vi "ch0 power normalization.vi"(1 "% of max":dbl=0.63, 2 "Gain":fxp<+,32,4>[](array[numeric]), 3 "Wave freq":fxp<+/-,64,32>[](array[numeric])) -> (0 "Array":fxp<+,32,2>[](array[numeric]))   [LabVIEW 2020]
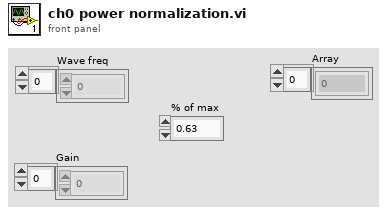
[diagram p1: front panel]
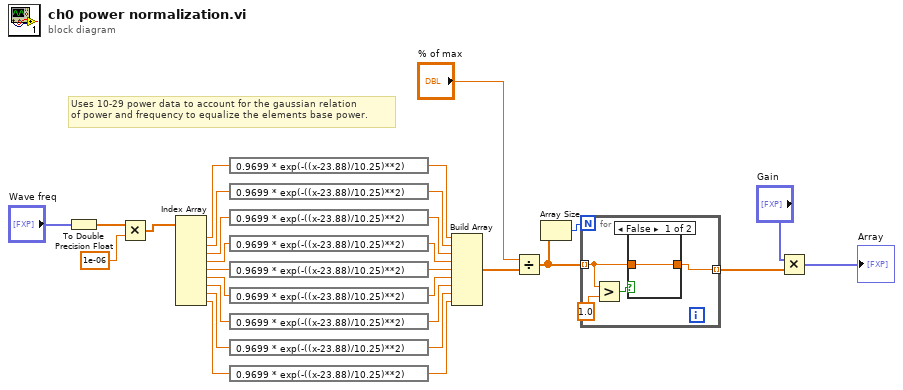
[diagram p0: block diagram]
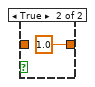
[diagram p2: hidden frame]
diagram:
  # "Uses 10-29 power data to account for the gaussian relation\nof power and frequency to equalize the elements base power."
  n1 = To Double Precision Float(number="Wave freq") -> (double precision float=w5:dbl[])
  n2 = Multiply(x=w5, y=1e-06) -> (x*y=w6:dbl[])
  n3 = Index Array(array=w6) -> (element #1=w9:dbl, element #2=w10:dbl, element #3=w11:dbl, element #4=w12:dbl, element #5=w13:dbl, element #6=w14:dbl, element #7=w15:dbl, element #8=w16:dbl, element #9=w17:dbl)  [unwired: 9 in]
  n4 = expression code="0.9699 * exp(-((x-23.88)/10.25)**2)"(w9) -> (w18:dbl)
  n5 = expression code="0.9699 * exp(-((x-23.88)/10.25)**2)"(w10) -> (w19:dbl)
  n6 = expression code="0.9699 * exp(-((x-23.88)/10.25)**2)"(w11) -> (w20:dbl)
  n7 = expression code="0.9699 * exp(-((x-23.88)/10.25)**2)"(w12) -> (w21:dbl)
  n8 = expression code="0.9699 * exp(-((x-23.88)/10.25)**2)"(w13) -> (w22:dbl)
  n9 = expression code="0.9699 * exp(-((x-23.88)/10.25)**2)"(w14) -> (w23:dbl)
  n10 = expression code="0.9699 * exp(-((x-23.88)/10.25)**2)"(w15) -> (w24:dbl)
  n11 = expression code="0.9699 * exp(-((x-23.88)/10.25)**2)"(w16) -> (w25:dbl)
  n12 = expression code="0.9699 * exp(-((x-23.88)/10.25)**2)"(w17) -> (w26:dbl)
  n13 = Build Array(w18, w19, w20, w21, w22, w23, w24, w25, w26) -> (w27:dbl[])
  n14 = Divide(x="% of max", y=w27) -> (x/y=w2:dbl[])
  n15 = Array Size(array=w2) -> (size(s)=w3:i32)
  n16 = for {
    N: w3 -> [_]
    tunnel: w2 -> [w31] mode=indexing
    tunnel: [w30] -> w1 mode=indexing
    n17 = Greater?(x=w31, y=1.0) -> (0:w32:bool)
    n18 = case shown="False" w32 {
      tunnel: [w34 1.0] -> w30
      tunnel: w31 -> [w34 _]
      frame False {
      }
      frame True {
      }
    }
  }
  n19 = Multiply(x="Gain", y=w1) -> (x*y=→"Array":fxp<+,32,2>[])
